vi "Lvi Get Board Names.vi"(8 "error in (no error)":errorcluster, 11 "BoardNumber":u32) -> (0 "error out":errorcluster, 1 "function return":u32(ring), 2 "BoardName":string, 3 "NumBoardsFound":u32)   [LabVIEW 2022 SP3, in "DtLvLink.lvlib"]
doc: "Calls directly into the entry points of the DLL of the Data Acq SDK to return name of the device. This VI is used by the higher-level VI, DtOLGetBoardNames."
uses:
  DtLvLink.lvlib
  <userlib>/LV-Link3/DtLvLink_64.dll
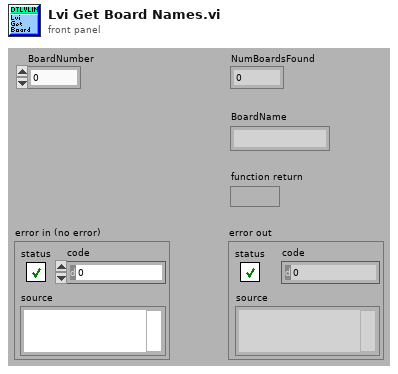
[diagram p1: front panel]
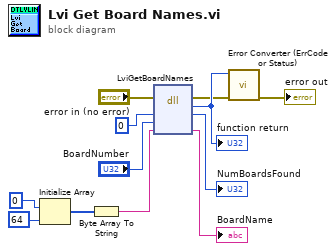
[diagram p0: block diagram]
diagram:
  n1 = Initialize Array(u8 0 ("element"), 64 ("dimension size")) -> (w8:u8[])
  n2 = Byte Array To String(unsigned byte array=w8) -> (string=w7:string)
  n3 = dll-call lib="C:/Program Files/National Instruments/LabVIEW 2022/user.lib/LV-Link3/DtLvLink_64.*" fn="LviGetBoardNames"(error in="error in (no error)", "NumBoardsFound"=u32 0, "BoardNumber"="BoardNumber", "BoardName"=w7) -> (error out=w2:errorcluster, w12:u32, "NumBoardsFound"=→"NumBoardsFound":u32, "BoardName"=→"BoardName":string)  [unwired: 3 in, 1 out]
  "function return" <- w12
  n4 = call "Error Converter (ErrCode or Status).vi"("error in (no error)"=w2, "error code"=w12) -> ("error out"=→"error out":errorcluster)  [unwired: 9 in]
